vi "Read Array of Observers.vi"(8 "error in (no error)":errorcluster, 11 "ObserverSet.lvclass in":refnum<class "ObserverSet.lvclass">) -> (0 "error out":errorcluster, 2 "Array of Observers":refnum<class "Send.lvclass">[](array[class]), 3 "ObserverSet.lvclass out":refnum<class "ObserverSet.lvclass">)   [LabVIEW 2011, in "Messenging.lvlib" / "ObserverSet.lvclass"]
uses:
  ObserverSet.lvclass
  Send/Send.lvclass
  ObserverSet.lvclass/ObserverSet.ctl
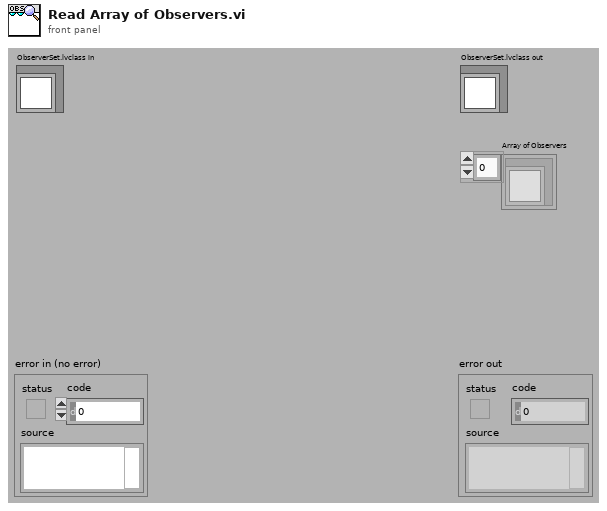
[diagram p1: front panel]
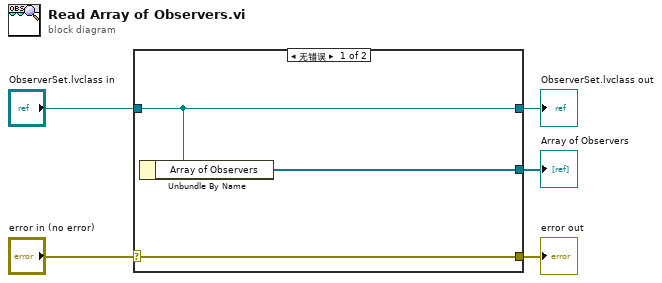
[diagram p0: block diagram]
diagram:
  n1 = case shown="无错误" "error in (no error)" {
    selector: "error in (no error)" -> [w8 w9]
    tunnel: [w8 w9] -> w4
    tunnel: [w7 w10] -> w2
    tunnel: "ObserverSet.lvclass in" -> [w7 w10]
    tunnel: [w6 _] -> w1
    frame No Error {
      n2 = Unbundle By Name(w7) -> ("Array of Observers"=w6:refnum<class "Send.lvclass">[])
    }
    frame Error {
    }
  }
  "error out" <- w4
  "ObserverSet.lvclass out" <- w2
  "Array of Observers" <- w1
